vi "add.vi"(0 "reference":refnum<class "SequenceDiagramGraph.lvclass">, 1 "node":refnum<class "AbstractNode.lvclass">, 2 "point":T1 {"y" format="%.2f"; "x" format="%.2f"}, 5 "error in (no error)":errorcluster) -> (14 "reference out":refnum<class "SequenceDiagramGraph.lvclass">, 15 "added":bool, 19 "error out":errorcluster)   [LabVIEW 2012, in "SequenceDiagramGraph.lvclass"]
doc: "public boolean add(Node n, Point2D p)"
uses:
  <resource>/Framework/Providers/Open_GDS/UML/SequenceDiagramGraph_class/SequenceDiagramGraph.lvclass
  <resource>/Framework/Providers/Open_GDS/UML/AbstractNode_class/AbstractNode.lvclass
  <resource>/Framework/Providers/Open_GDS/UML/General/Point/Point Point2D.ctl
  <resource>/Framework/Providers/Open_GDS/UML/CallNode_class/CallNode.lvclass
  <resource>/Framework/Providers/Open_GDS/UML/Graph_class/Graph.lvclass
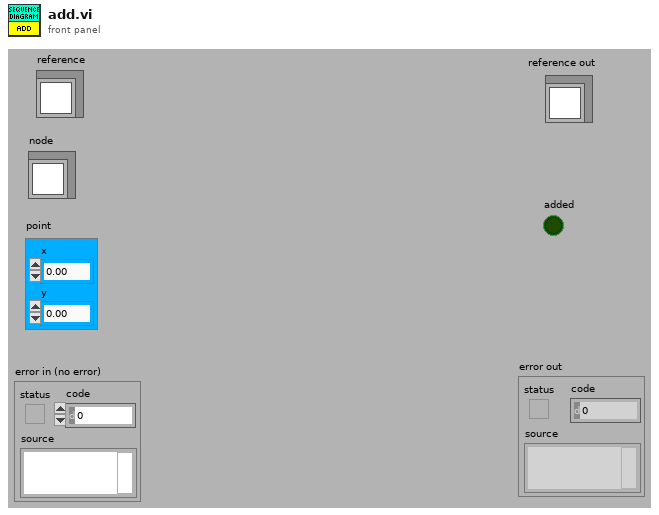
[diagram p1: front panel]
types:
  T1 = typedef "Point Point2D.ctl" = cluster{"x":dbl, "y":dbl}
  T2 = typedef "SequenceDiagramGraph.lvclass/ObjectAttributes.ctl" = cluster{"Base class":T3, "none":bool}
  T3 = typedef "Graph.lvclass/ObjectAttributes.ctl" = cluster{"nodes":refnum<class "AbstractNode.lvclass">[], "edges":refnum<class "AbstractEdge.lvclass">[], "nodesToBeRemoved":refnum<class "AbstractNode.lvclass">[], "edgesToBeRemoved":refnum<class "AbstractEdge.lvclass">[], "needsLayout":bool, "LayoutNodes":refnum<class "AbstractNode.lvclass">[]}
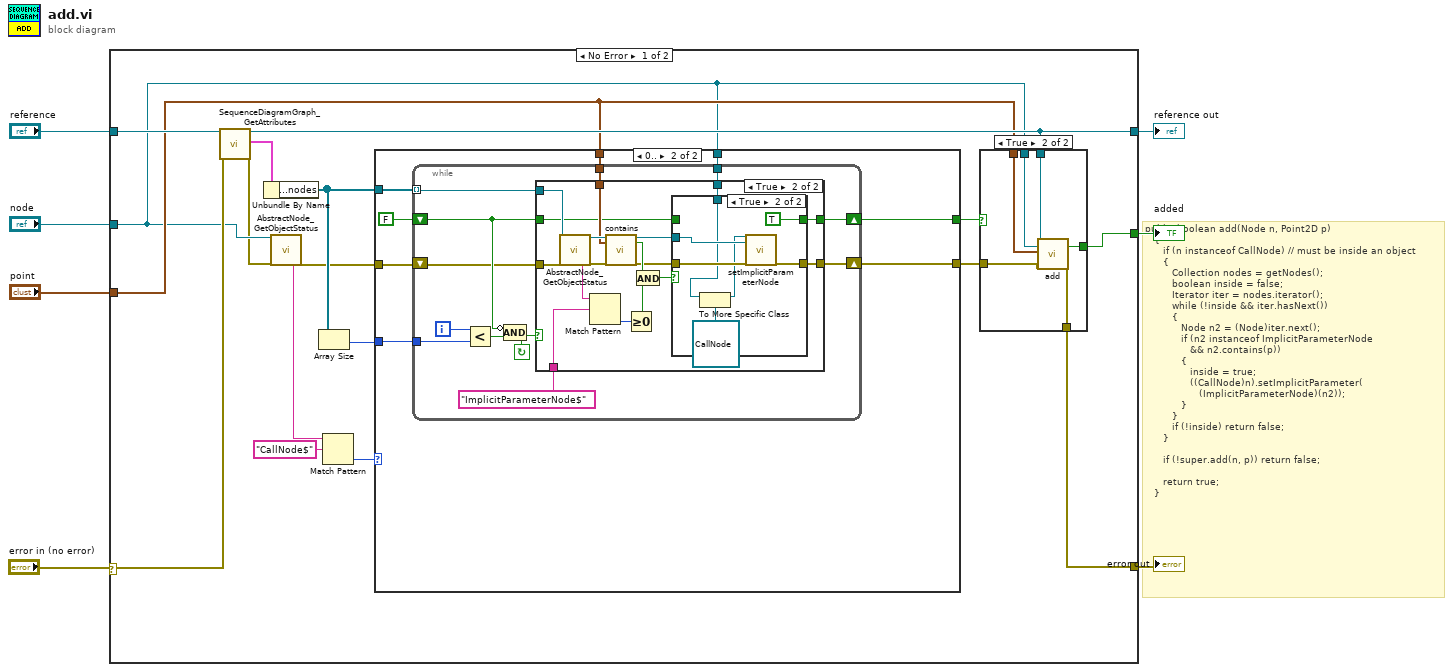
[diagram p0: block diagram]
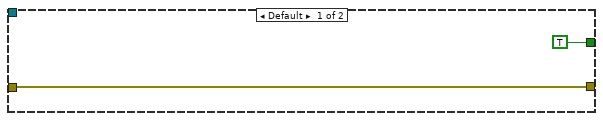
[diagram p3: hidden frame]
diagram:
  # "public boolean add(Node n, Point2D p)\n   {\n      if (n instanceof CallNode) // must be inside an object\n      {\n         Collection nodes = getNodes();\n         boolean inside = false;\n         Iterator iter = nodes.iterator();\n         while (!inside && iter.hasNext())\n         {\n            Node n2 = (Node)iter.next();\n            if (n2 instanceof ImplicitParameterNode\n               && n2.contains(p)) \n            {\n               inside = true;\n               ((CallNode)n).setImplicitParameter(\n                  (ImplicitParameterNode)(n2));\n            }\n         }\n         if (!inside) return false;\n      }\n\n      if (!super.add(n, p)) return false;\n\n      return true;\n   }"
  n1 = case shown="No Error" "error in (no error)" {
    selector: "error in (no error)" -> [w21 w83]
    tunnel: "reference" -> [w24 w84]
    tunnel: [w23 w83] -> w6
    tunnel: [w22 w84] -> w5
    tunnel: "node" -> [w18 _]
    tunnel: "point" -> [w19 _]
    tunnel: [w20 _] -> w1
    frame No Error {
      n2 = call <resource>:"SequenceDiagramGraph_GetAttributes.vi"("reference in"=w24, "error in (no error)"=w21) -> ("reference out"=w22:refnum<class "SequenceDiagramGraph.lvclass">, "Attributes"=w17:T2, "error out"=w13:errorcluster)  [unwired: 15 out]
      n3 = Unbundle By Name(w17) -> ("Base class.nodes"=w12:refnum<class "AbstractNode.lvclass">[])
      n4 = call <resource>:"AbstractNode_GetObjectStatus.vi"("reference in"=w18, "error in (no error)"=w13) -> ("Class name"=w16:string, "error out"=w9:errorcluster)  [unwired: 16 out]
      n5 = Array Size(array=w12) -> (size(s)=w11:i32)
      n6 = Match Pattern(string=w16, regular expression="CallNode$") -> (offset past match=w14:i32)  [unwired: 4 out]
      n7 = case shown="0.." w14 {
        tunnel: w12 -> [_ w41]
        tunnel: w11 -> [_ w40]
        tunnel: w19 -> [_ w39]
        tunnel: [TRUE w38] -> w10
        tunnel: w18 -> [_ w37]
        tunnel: w9 -> [w34 w35]
        tunnel: [w34 w36] -> w8
        frame Default {
        }
        frame 0.. {
          n8 = while {
            shift-right: [w49] -> w38
            shift-left: FALSE -> [w50]
            tunnel: w41 -> [w48] mode=indexing
            tunnel: w40 -> [w53]
            tunnel: w39 -> [w46]
            tunnel: w37 -> [w45]
            shift-right: [w44] -> w36
            shift-left: w35 -> [w43]
            i -> [w54]
            stop <- w51 continue-if-true
            n9 = Less?(x=w54, y=w53) -> (x < y?=w52:bool)
            n10 = Compound Arithmetic op=AND(invert w50, w52) -> (w51:bool)
            n11 = case shown="True" w51 {
              tunnel: w50 -> [w56 w63]
              tunnel: [w56 w62] -> w49
              tunnel: w48 -> [_ w73]
              tunnel: "ImplicitParameterNode$" ("regular expression") -> [_ w71]
              tunnel: w46 -> [_ w67]
              tunnel: w45 -> [_ w59]
              tunnel: w43 -> [w55 w58]
              tunnel: [w55 w57] -> w44
              frame False {
              }
              frame True {
                n12 = call <resource>:"AbstractNode_GetObjectStatus.vi"("reference in"=w73, "error in (no error)"=w58) -> ("Class name"=w72:string, "reference out"=w69:refnum<class "AbstractNode.lvclass">, "error out"=w68:errorcluster)  [unwired: 15 out]
                n13 = Match Pattern(string=w72, regular expression=w71) -> (offset past match=w70:i32)  [unwired: 4 out]
                n14 = call-dynamic "contains.vi"("reference"=w69, "point2D"=w67, "error in (no error)"=w68) -> ("reference out"=w60:refnum<class "AbstractNode.lvclass">, "contains"=w65:bool, "error out"=w61:errorcluster)  [unwired: 14 in]
                n15 = Greater Or Equal To 0?(x=w70) -> (x >= 0?=w64:bool)
                n16 = And(x=w65, y=w64) -> (x .and. y?=w66:bool)
                n17 = case shown="True" w66 {
                  tunnel: w63 -> [w75 _]
                  tunnel: [w75 TRUE] -> w62
                  tunnel: w61 -> [w74 w81]
                  tunnel: w60 -> [_ w80]
                  tunnel: w59 -> [_ w78]
                  tunnel: [w74 w79] -> w57
                  frame False {
                  }
                  frame True {
                    n18 = To More Specific Class(target class=refnum<class "CallNode.lvclass"> refnum ("reference"), reference=w78) -> (specific class reference=w76:refnum<class "CallNode.lvclass">)  [unwired: 1 in, 1 out]
                    n19 = call-dynamic "setImplicitParameterNode.vi"("reference"=w76, "objectCallNodeRef"=w80, "error in (no error)"=w81) -> ("error out"=w79:errorcluster)  [unwired: 15 in, 1 out]
                  }
                }
              }
            }
          }
        }
      }
      n20 = case shown="True" w10 {
        selector: w10 -> [w26 _]
        tunnel: w18 -> [_ w31]
        tunnel: [w26 w27] -> w20
        tunnel: [w25 w28] -> w23
        tunnel: w19 -> [_ w30]
        tunnel: w8 -> [w25 w29]
        tunnel: w22 -> [_ w32]
        frame False {
        }
        frame True {
          n21 = call-parent "add.vi"("reference"=w32, "node"=w31, "point"=w30, "error in (no error)"=w29) -> ("added"=w27:bool, "error out"=w28:errorcluster)  [unwired: 13 in, 1 out]
        }
      }
    }
    frame Error {
    }
  }
  "reference out" <- w5
  "error out" <- w6
  "added" <- w1
